vi "test-SwerveModulePosition.vi"(8 "error in (no error)":errorcluster) -> (0 "error out":errorcluster, 3 "ALL TESTS PASSED":bool)   [LabVIEW 2019]
uses:
  <vilib>/Rock Robotics/WPI/ThirdParty/JAS_Junk/TrajLib/Rotation2d_Minus.vi
  <vilib>/Rock Robotics/WPI/ThirdParty/JAS_Junk/TrajLib/Rotation2d_GetRadians.vi
  <vilib>/Rock Robotics/WPI/ThirdParty/JAS_Junk/TrajLib/Rotation2d_RotateBy.vi
  <vilib>/Rock Robotics/WPI/ThirdParty/JAS_Junk/TrajLib/Rotation2d_UnaryMinus.vi
  <vilib>/Rock Robotics/WPI/ThirdParty/JAS_Junk/TrajLib/Rotation2d_CreateXY.vi
  <vilib>/Rock Robotics/WPI/ThirdParty/JAS_Junk/TrajLib/Util_CalcDist.vi
  <vilib>/Rock Robotics/WPI/ThirdParty/JAS_Junk/TrajLib/Trajectory_Library.lvlib
panel:
  out "Test 2":bool
  out "Test 1":bool
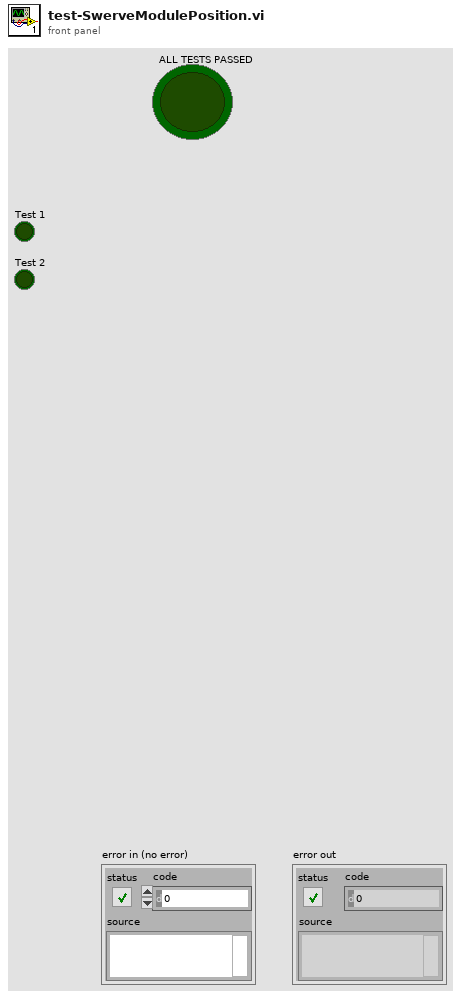
[diagram p1: front panel]
types:
  T1 = typedef "Trajectory_Library.lvlib/ROTATION2D.ctl" = cluster{"VALUE":dbl, "COS":dbl, "SIN":dbl}
  T2 = typedef "Trajectory_Library.lvlib/SWERVE_DRIVE_MODULE_POSITION.ctl" = cluster{"Distance":dbl, "Angle":T1, "P":bool}
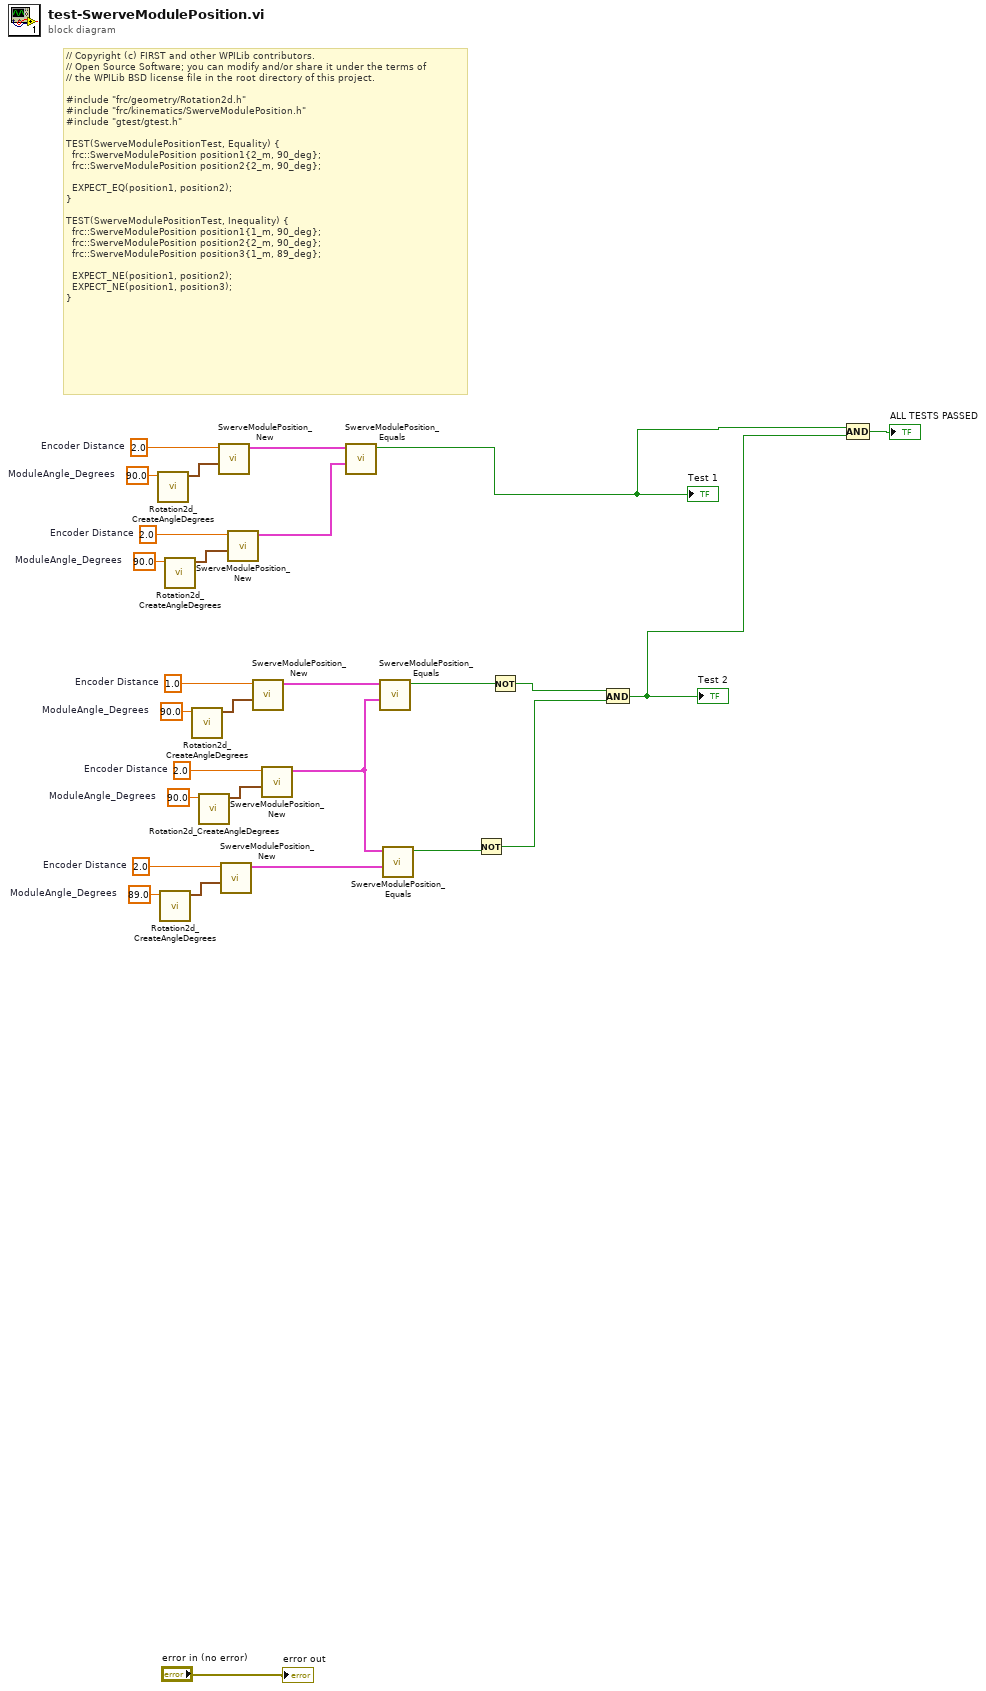
[diagram p0: block diagram]
diagram:
  w8 = 2.0  # Encoder Distance
  w7 = 89.0  # ModuleAngle_Degrees
  w14 = 2.0  # Encoder Distance
  w13 = 1.0  # Encoder Distance
  w12 = 90.0  # ModuleAngle_Degrees
  w11 = 90.0  # ModuleAngle_Degrees
  w23 = 2.0  # Encoder Distance
  w22 = 2.0  # Encoder Distance
  w21 = 90.0  # ModuleAngle_Degrees
  w20 = 90.0  # ModuleAngle_Degrees
  # "// Copyright (c) FIRST and other WPILib contributors.\n// Open Source Software; you can modify and/or share it under the terms of\n// the WPILib BSD license file in the root directory of this project.\n\n#include \"frc/geometry/Rotation2d.h\"\n#include \"frc/kinematics/SwerveModulePosition.h\"\n#include \"gtest/gtest.h\"\n\nTEST(SwerveModulePositionTest, Equality) {\n  frc::SwerveModulePosition position1{2_m, 90_deg};\n  frc::SwerveModulePosition position2{2_m, 90_deg};\n\n  EXPECT_EQ(position1, position2);\n}\n\nTEST(SwerveModulePositionTest, Inequality) {\n  frc::SwerveModulePosition position1{1_m, 90_deg};\n  frc::SwerveModulePosition position2{2_m, 90_deg};\n  frc::SwerveModulePosition position3{1_m, 89_deg};\n\n  EXPECT_NE(position1, position2);\n  EXPECT_NE(position1, position3);\n}"
  n1 = call <vilib>:"Rotation2d_CreateAngleDegrees.vi"("Angle_Degrees"=w20) -> ("ROTATION"=w24:T1)  [unwired: 10 in]
  n2 = call <vilib>:"Rotation2d_CreateAngleDegrees.vi"("Angle_Degrees"=w7) -> ("ROTATION"=w9:T1)  [unwired: 10 in]
  n3 = call <vilib>:"Rotation2d_CreateAngleDegrees.vi"("Angle_Degrees"=w21) -> ("ROTATION"=w25:T1)  [unwired: 10 in]
  n4 = call <vilib>:"Rotation2d_CreateAngleDegrees.vi"("Angle_Degrees"=w11) -> ("ROTATION"=w15:T1)  [unwired: 10 in]
  n5 = call <vilib>:"Rotation2d_CreateAngleDegrees.vi"("Angle_Degrees"=w12) -> ("ROTATION"=w16:T1)  [unwired: 10 in]
  n6 = call <vilib>:"SwerveModulePosition_New.vi"("ROTATION"=w24, "Distance"=w22) -> ("SWERVE_DRIVE_MODULE_POSITION"=w19:T2)  [unwired: 9 in]
  n7 = call <vilib>:"SwerveModulePosition_New.vi"("ROTATION"=w9, "Distance"=w8) -> ("SWERVE_DRIVE_MODULE_POSITION"=w6:T2)  [unwired: 9 in]
  n8 = call <vilib>:"SwerveModulePosition_New.vi"("ROTATION"=w25, "Distance"=w23) -> ("SWERVE_DRIVE_MODULE_POSITION"=w18:T2)  [unwired: 9 in]
  n9 = call <vilib>:"SwerveModulePosition_New.vi"("ROTATION"=w15, "Distance"=w13) -> ("SWERVE_DRIVE_MODULE_POSITION"=w10:T2)  [unwired: 9 in]
  n10 = call <vilib>:"SwerveModulePosition_New.vi"("ROTATION"=w16, "Distance"=w14) -> ("SWERVE_DRIVE_MODULE_POSITION"=w5:T2)  [unwired: 9 in]
  n11 = call <vilib>:"SwerveModulePosition_Equals.vi"("other SWERVE_DRIVE_MODULE_POSITION"=w18, "in SWERVE_DRIVE_MODULE_POSITION"=w19) -> ("Equals"=w17:bool)  [unwired: 9 in]
  "Test 1" <- w17
  n12 = call <vilib>:"SwerveModulePosition_Equals.vi"("other SWERVE_DRIVE_MODULE_POSITION"=w5, "in SWERVE_DRIVE_MODULE_POSITION"=w10) -> ("Equals"=w1:bool)  [unwired: 9 in]
  n13 = call <vilib>:"SwerveModulePosition_Equals.vi"("other SWERVE_DRIVE_MODULE_POSITION"=w6, "in SWERVE_DRIVE_MODULE_POSITION"=w5) -> ("Equals"=w4:bool)  [unwired: 9 in]
  n14 = Not(x=w4) -> (.not. x?=w3:bool)
  n15 = Not(x=w1) -> (.not. x?=w2:bool)
  n16 = And(x=w2, y=w3) -> (x .and. y?=w28:bool)
  "Test 2" <- w28
  n17 = Compound Arithmetic op=AND(w17, w28) -> (→"ALL TESTS PASSED":bool)
  "error out" <- "error in (no error)"
